vi "Consume Materials.vi"(0 "Factory Status in":T3, 1 "Materials":T1[](array[typedef]) {"Mineral" items=["Ore", "Clay", "Obsidian", "Geode", "Open Geode"]}) -> (2 "Factory Status out":T3)   [LabVIEW 2020, in "AoC 2022.lvlib"]
uses:
  AoC 2022.lvlib
  Mineral_Enum.ctl
  Inventory.ctl
  Robot Factory.ctl
  Step.ctl
  Mineral.ctl
  Cost.ctl
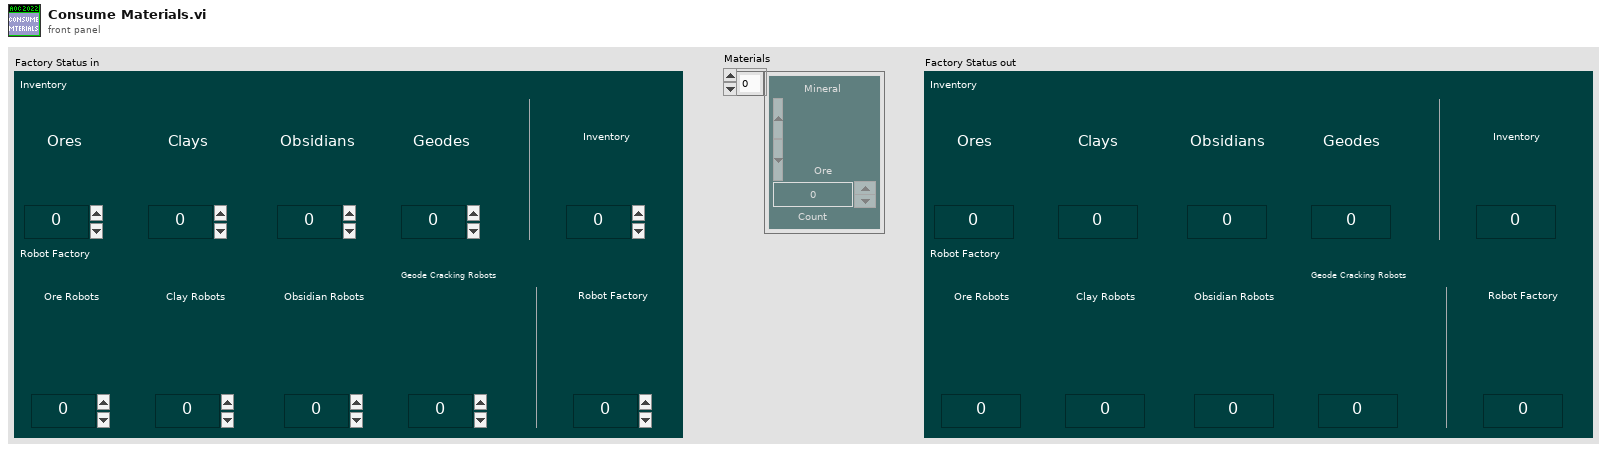
[diagram p1: front panel]
types:
  T1 = typedef "AoC 2022.lvlib/Cost.ctl" = cluster{"Mineral":T2, "Count":u32}
  T2 = typedef "AoC 2022.lvlib/Mineral.ctl" = u16
  T3 = typedef "AoC 2022.lvlib/Step.ctl" = cluster{"Inventory":T4, "Robot Factory":T5}
  T4 = typedef "AoC 2022.lvlib/Inventory.ctl" = cluster{"Ores":u32, "Clays":u32, "Obsidians":u32, "Geodes":u32, "Inventory":u32}
  T5 = typedef "AoC 2022.lvlib/Robot Factory.ctl" = cluster{"Ore Robots":u32, "Clay Robots":u32, "Obsidian Robots":u32, "Geode Cracking Robots":u32, "Robot Factory":u32}
  T6 = typedef "AoC 2022.lvlib/Mineral_Enum.ctl" = enum16{"ore", "clay", "obsidian", "geode", "Open Geode"}
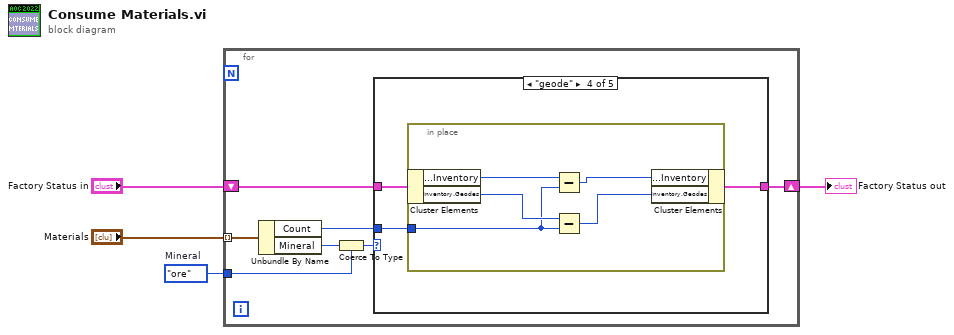
[diagram p0: block diagram]
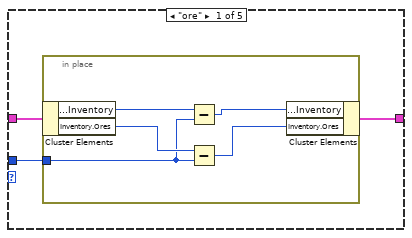
[diagram p2: hidden frame]
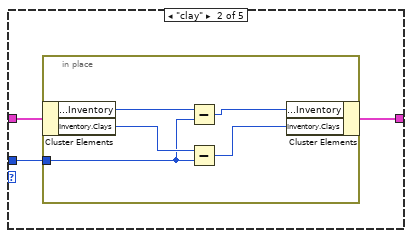
[diagram p3: hidden frame]
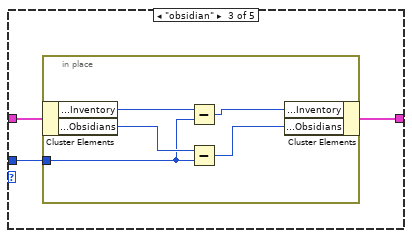
[diagram p4: hidden frame]
diagram:
  w3 = Mineral_Enum."ore"  # Mineral
  n1 = for {
    tunnel: "Materials" -> [w10] mode=indexing
    shift-right: [w5] -> w4
    shift-left: "Factory Status in" -> [w11]
    tunnel: w3 -> [w7]
    n2 = Unbundle By Name(w10) -> ("Count"=w9:u32, "Mineral"=w8:T2)
    n3 = Coerce To Type(0:w8, 1:w7) -> (2:w6:T6)
    n4 = case shown="\"geode\"" w6 {
      tunnel: w11 -> [w14 w22 w30 w38 w44]
      tunnel: w9 -> [w13 w21 w29 w37 _]
      tunnel: [w12 w20 w28 w36 w44] -> w5
      frame "ore" {
        n5 = in-place {
          in-place-border: w13 -> [w15]
          n6 = in-place-cluster #1(w14) -> ("Inventory.Inventory"=w17:u32, "Inventory.Ores"=w19:u32)
          n7 = Subtract(x=w17, y=w15) -> (x-y=w16:u32)
          n8 = Subtract(x=w19, y=w15) -> (x-y=w18:u32)
          n9 = in-place-cluster #1("Inventory.Inventory"=w16, "Inventory.Ores"=w18) -> (w12:T3)
        }
      }
      frame "clay" {
        n10 = in-place {
          in-place-border: w21 -> [w23]
          n11 = in-place-cluster #2(w22) -> ("Inventory.Inventory"=w25:u32, "Inventory.Clays"=w27:u32)
          n12 = Subtract(x=w25, y=w23) -> (x-y=w24:u32)
          n13 = Subtract(x=w27, y=w23) -> (x-y=w26:u32)
          n14 = in-place-cluster #2("Inventory.Inventory"=w24, "Inventory.Clays"=w26) -> (w20:T3)
        }
      }
      frame "obsidian" {
        n15 = in-place {
          in-place-border: w29 -> [w31]
          n16 = in-place-cluster #3(w30) -> ("Inventory.Inventory"=w33:u32, "Inventory.Obsidians"=w35:u32)
          n17 = Subtract(x=w33, y=w31) -> (x-y=w32:u32)
          n18 = Subtract(x=w35, y=w31) -> (x-y=w34:u32)
          n19 = in-place-cluster #3("Inventory.Inventory"=w32, "Inventory.Obsidians"=w34) -> (w28:T3)
        }
      }
      frame "geode" {
        n20 = in-place {
          in-place-border: w37 -> [w39]
          n21 = in-place-cluster #4(w38) -> ("Inventory.Inventory"=w41:u32, "Inventory.Geodes"=w43:u32)
          n22 = Subtract(x=w41, y=w39) -> (x-y=w40:u32)
          n23 = Subtract(x=w43, y=w39) -> (x-y=w42:u32)
          n24 = in-place-cluster #4("Inventory.Inventory"=w40, "Inventory.Geodes"=w42) -> (w36:T3)
        }
      }
      frame "Open Geode" {
      }
    }
  }
  "Factory Status out" <- w4
